vi "Drift_Compensator.vi"(7 "Device Number":T1, 9 "Zero Yaw":bool, 11 "Raw Yaw":dbl) -> (3 "comp yaw":dbl format="%#.1f")   [LabVIEW 2016, in "navX Library.lvlib"]
uses:
  navX Library.lvlib
  _TypeDefs/FRIC_navX_DeviceNumbersTypeDef.ctl
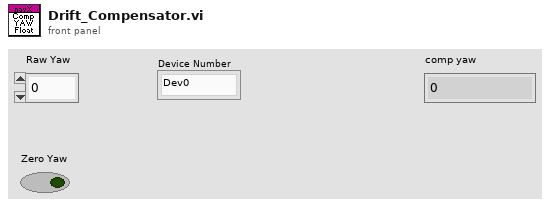
[diagram p1: front panel]
types:
  T1 = typedef "navX Library.lvlib/FRIC_navX_DeviceNumbersTypeDef.ctl" = enum16{"Dev0", "Dev1", "Dev2", "Dev3"}
  T2 = cluster{"current time":u32, "Error":dbl, "Drift error":dbl}
  T3 = cluster{"current time":u32, "Error":dbl, "Drift error":dbl}[]
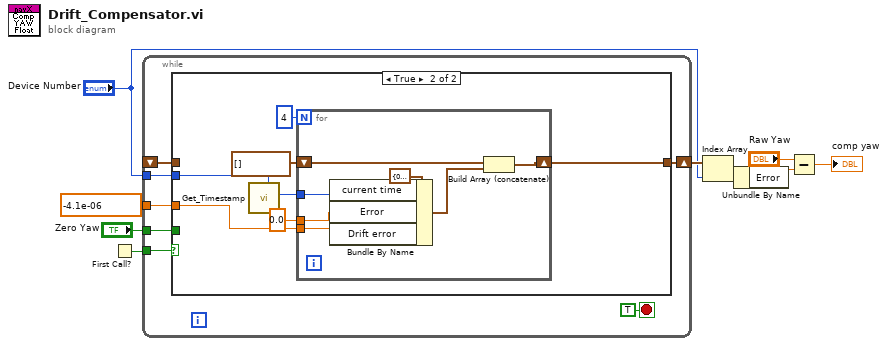
[diagram p0: block diagram]
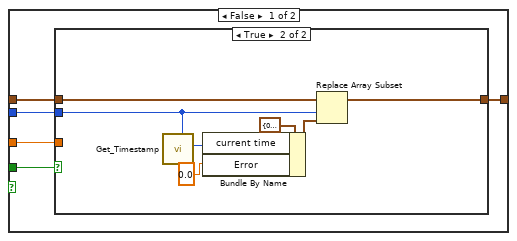
[diagram p2: hidden frame]
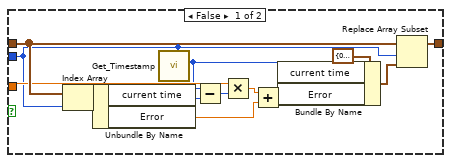
[diagram p3: hidden frame]
diagram:
  n1 = First Call?() -> (First Call?: T/F=w7:bool)
  n2 = while {
    shift-right: [w13] -> w5
    shift-left: _ -> [w12]
    tunnel: "Zero Yaw" -> [w15]
    tunnel: w7 -> [w14]
    tunnel: "Device Number" -> [w11]
    tunnel: -4.1e-06 ("Dev0 Drift K/sec") -> [w10]
    stop <- TRUE stop-if-true
    n3 = case shown="True" w14 {
      tunnel: w15 -> [w21 _]
      tunnel: [w18 w47] -> w13
      tunnel: w12 -> [w20 _]
      tunnel: w11 -> [w19 w42]
      tunnel: w10 -> [w17 w46]
      frame False {
        n4 = case shown="True" w21 {
          tunnel: w20 -> [w31 w41]
          tunnel: w19 -> [w22 w35]
          tunnel: [w30 w40] -> w18
          tunnel: w17 -> [w26 _]
          frame False {
            n5 = Index Array(array=w31, index=w22) -> (element=w33:T2)
            n6 = Unbundle By Name(w33) -> ("current time"=w32:u32, "Error"=w24:dbl)
            n7 = call "Get_Timestamp.vi"("Device Number"=w22) -> ("Timestamp"=w23:u32)  [unwired: 10 in]
            n8 = Subtract(x=w23, y=w32) -> (x-y=w34:u32)
            n9 = Multiply(x=w26, y=w34) -> (x*y=w25:dbl)
            n10 = Add(x=w25, y=w24) -> (x+y=w27:dbl)
            n11 = Bundle By Name(cluster=T2 {"current time"=0, "Error"=0.0, "Drift error"=0.0} ("new element/subarray"), "current time"=w23, "Error"=w27) -> (w28:T2)
            n12 = Replace Array Subset(array=w31, new element=w28, index=w22) -> (w30:T3)
          }
          frame True {
            n13 = call "Get_Timestamp.vi"("Device Number"=w35) -> ("Timestamp"=w36:u32)  [unwired: 10 in]
            n14 = Bundle By Name(cluster=T2 {"current time"=0, "Error"=0.0, "Drift error"=0.0} ("new element/subarray"), "current time"=w36, "Error"=0.0) -> (w38:T2)
            n15 = Replace Array Subset(array=w41, new element=w38, index=w35) -> (w40:T3)
          }
        }
      }
      frame True {
        n16 = call "Get_Timestamp.vi"("Device Number"=w42) -> ("Timestamp"=w43:u32)  [unwired: 10 in]
        n17 = for {
          N: 4 ("dimension size") -> [_]
          tunnel: w43 -> [w54]
          shift-right: [w51] -> w47
          shift-left: T3 [] -> [w53]
          tunnel: w46 -> [w50]
          tunnel: 0.0 ("Error") -> [w49]
          n18 = Bundle By Name(cluster=T2 {"current time"=0, "Error"=0.0, "Drift error"=-0.004447}, "current time"=w54, "Error"=w49, "Drift error"=w50) -> (w52:T2)
          n19 = Build Array (concatenate)(w53, w52) -> (w51:T3)
        }
      }
    }
  }
  n20 = Index Array(array=w5, index="Device Number") -> (element=w3:T2)
  n21 = Unbundle By Name(w3) -> ("Error"=w2:dbl)
  n22 = Subtract(x="Raw Yaw", y=w2) -> (x-y=→"comp yaw":dbl)
